vi "niFPGA Sine Wave Generator.vi"(1 "reset":bool) -> (4 "sine out":i16)   [LabVIEW 2017]
doc: "Generates a point-by-point sine wave using direct digital synthesis. The synthesis runs continuously from the top-level FPGA target clock to produce an accurate real-time frequency. Each execution of this VI returns the most recent sample produced by the underlying synthesis engine."
panel:
  out "cosine out":i16
  in  "phase offset (periods)":fxp<+,32,0>
  in  "frequency (periods/tick)":fxp<+,32,0>=0.9999999997671694
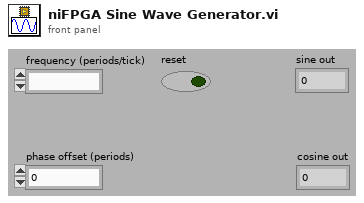
[diagram p1: front panel]
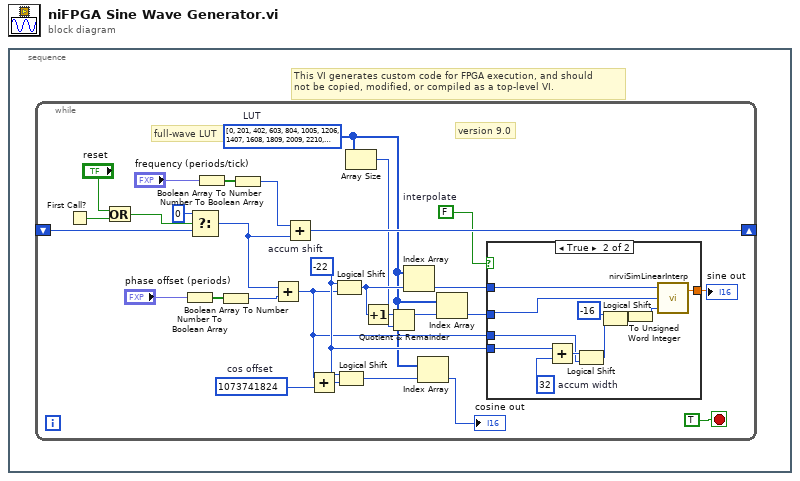
[diagram p0: block diagram]
diagram:
  n1 = stacked-sequence {
    frame #0 {
      # "This VI generates custom code for FPGA execution, and should\nnot be copied, modified, or compiled as a top-level VI."
      n2 = while {
        shift-right: [w28] -> _
        shift-left: _ -> [w18]
        stop <- TRUE stop-if-true
        w1 = u32 1073741824  # cos offset
        w8 = i32[] [0, 201, 402, 603, 804, 1005, 1206, 1407, 1608, 1809, 2009, 2210, 2411, 2611, 2811, 3012, 3212, 3412, 3612, 3811, 4011, 4211, 4410, 4609, 4808, 5007, 5205, 5404, 5602, 5800, 5998, 6195, 6393, 6590, 6787, 6983, 7179, 7375, 7571, 7767, 7962, 8157, 8351, 8546, 8740, 8933, 9126, 9319, 9512, 9704, 9896, 10087, 10279, 10469, 10660, 10850, 11039, 11228, 11417, 11605, 11793, 11980, 12167, 12354, 12540, 12725, 12910, 13095, 13279, 13462, 13645, 13828, 14010, 14191, 14372, 14553, 14733, 14912, 15091, 15269, 15446, 15624, 15800, 15976, 16151, 16326, 16500, 16673, 16846, 17018, 17189, 17360, 17531, 17700, 17869, 18037, 18205, 18371, 18538, 18703, 18868, 19032, 19195, 19358, 19520, 19681, 19841, 20001, 20160, 20318, 20475, 20632, 20787, 20943, 21097, 21250, 21403, 21555, 21706, 21856, 22005, 22154, 22302, 22448, 22595, 22740, 22884, 23028, 23170, 23312, 23453, 23593, 23732, 23870, 24007, 24144, 24279, 24414, 24547, 24680, 24812, 24943, 25073, 25202, 25330, 25457, 25583, 25708, 25832, 25955, 26078, 26199, 26319, 26438, 26557, 26674, 26790, 26905, 27020, 27133, 27245, 27356, 27467, 27576, 27684, 27791, 27897, 28002, 28106, 28208, 28310, 28411, 28511, 28609, 28707, 28803, 28898, 28993, 29086, 29178, 29269, 29359, 29447, 29535, 29621, 29707, 29791, 29874, 29956, 30037, 30117, 30196, 30273, 30350, 30425, 30499, 30572, 30644, 30714, 30784, 30852, 30919, 30985, 31050, 31114, 31176, 31237, 31298, 31357, 31414, 31471, 31526, 31581, 31634, 31685, 31736, 31785, 31834, 31881, 31927, 31971, 32015, 32057, 32098, 32138, 32177, 32214, 32250, 32285, 32319, 32351, 32383, 32413, 32442, 32469, 32496, 32521, 32545, 32568, 32589, 32610, 32629, 32647, 32663, 32679, 32693, 32706, 32718, 32728, 32737, 32745, 32752, 32758, 32762, 32765, 32767, 32767, 32767, 32765, 32762, 32758, 32752, 32745, 32737, 32728, 32718, 32706, 32693, 32679, 32663, 32647, 32629, 32610, 32589, 32568, 32545, 32521, 32496, 32469, 32442, 32413, 32383, 32351, 32319, 32285, 32250, 32214, 32177, 32138, 32098, 32057, 32015, 31971, 31927, 31881, 31834, 31785, 31736, 31685, 31634, 31581, 31526, 31471, 31414, 31357, 31298, 31237, 31176, 31114, 31050, 30985, 30919, 30852, 30784, 30714, 30644, 30572, 30499, 30425, 30350, 30273, 30196, 30117, 30037, 29956, 29874, 29791, 29707, 29621, 29535, 29447, 29359, 29269, 29178, 29086, 28993, 28898, 28803, 28707, 28609, 28511, 28411, 28310, 28208, 28106, 28002, 27897, 27791, 27684, 27576, 27467, 27356, 27245, 27133, 27020, 26905, 26790, 26674, 26557, 26438, 26319, 26199, 26078, 25955, 25832, 25708, 25583, 25457, 25330, 25202, 25073, 24943, 24812, 24680, 24547, 24414, 24279, 24144, 24007, 23870, 23732, 23593, 23453, 23312, 23170, 23028, 22884, 22740, 22595, 22448, 22302, 22154, 22005, 21856, 21706, 21555, 21403, 21250, 21097, 20943, 20787, 20632, 20475, 20318, 20160, 20001, 19841, 19681, 19520, 19358, 19195, 19032, 18868, 18703, 18538, 18371, 18205, 18037, 17869, 17700, 17531, 17360, 17189, 17018, 16846, 16673, 16500, 16326, 16151, 15976, 15800, 15624, 15446, 15269, 15091, 14912, 14733, 14553, 14372, 14191, 14010, 13828, 13645, 13462, 13279, 13095, 12910, 12725, 12540, 12354, 12167, 11980, 11793, 11605, 11417, 11228, 11039, 10850, 10660, 10469, 10279, 10087, 9896, 9704, 9512, 9319, 9126, 8933, 8740, 8546, 8351, 8157, 7962, 7767, 7571, 7375, 7179, 6983, 6787, 6590, 6393, 6195, 5998, 5800, 5602, 5404, 5205, 5007, 4808, 4609, 4410, 4211, 4011, 3811, 3612, 3412, 3212, 3012, 2811, 2611, 2411, 2210, 2009, 1809, 1608, 1407, 1206, 1005, 804, 603, 402, 201, 0, -201, -402, -603, -804, -1005, -1206, -1407, -1608, -1809, -2009, -2210, -2411, -2611, -2811, -3012, -3212, -3412, -3612, -3811, -4011, -4211, -4410, -4609, -4808, -5007, -5205, -5404, -5602, -5800, -5998, -6195, -6393, -6590, -6787, -6983, -7179, -7375, -7571, -7767, -7962, -8157, -8351, -8546, -8740, -8933, -9126, -9319, -9512, -9704, -9896, -10087, -10279, -10469, -10660, -10850, -11039, -11228, -11417, -11605, -11793, -11980, -12167, -12354, -12540, -12725, -12910, -13095, -13279, -13462, -13645, -13828, -14010, -14191, -14372, -14553, -14733, -14912, -15091, -15269, -15446, -15624, -15800, -15976, -16151, -16326, -16500, -16673, -16846, -17018, -17189, -17360, -17531, -17700, -17869, -18037, -18205, -18371, -18538, -18703, -18868, -19032, -19195, -19358, -19520, -19681, -19841, -20001, -20160, -20318, -20475, -20632, -20787, -20943, -21097, -21250, -21403, -21555, -21706, -21856, -22005, -22154, -22302, -22448, -22595, -22740, -22884, -23028, -23170, -23312, -23453, -23593, -23732, -23870, -24007, -24144, -24279, -24414, -24547, -24680, -24812, -24943, -25073, -25202, -25330, -25457, -25583, -25708, -25832, -25955, -26078, -26199, -26319, -26438, -26557, -26674, -26790, -26905, -27020, -27133, -27245, -27356, -27467, -27576, -27684, -27791, -27897, -28002, -28106, -28208, -28310, -28411, -28511, -28609, -28707, -28803, -28898, -28993, -29086, -29178, -29269, -29359, -29447, -29535, -29621, -29707, -29791, -29874, -29956, -30037, -30117, -30196, -30273, -30350, -30425, -30499, -30572, -30644, -30714, -30784, -30852, -30919, -30985, -31050, -31114, -31176, -31237, -31298, -31357, -31414, -31471, -31526, -31581, -31634, -31685, -31736, -31785, -31834, -31881, -31927, -31971, -32015, -32057, -32098, -32138, -32177, -32214, -32250, -32285, -32319, -32351, -32383, -32413, -32442, -32469, -32496, -32521, -32545, -32568, -32589, -32610, -32629, -32647, -32663, -32679, -32693, -32706, -32718, -32728, -32737, -32745, -32752, -32758, -32762, -32765, -32767, -32767, -32767, -32765, -32762, -32758, -32752, -32745, -32737, -32728, -32718, -32706, -32693, -32679, -32663, -32647, -32629, -32610, -32589, -32568, -32545, -32521, -32496, -32469, -32442, -32413, -32383, -32351, -32319, -32285, -32250, -32214, -32177, -32138, -32098, -32057, -32015, -31971, -31927, -31881, -31834, -31785, -31736, -31685, -31634, -31581, -31526, -31471, -31414, -31357, -31298, -31237, -31176, -31114, -31050, -30985, -30919, -30852, -30784, -30714, -30644, -30572, -30499, -30425, -30350, -30273, -30196, -30117, -30037, -29956, -29874, -29791, -29707, -29621, -29535, -29447, -29359, -29269, -29178, -29086, -28993, -28898, -28803, -28707, -28609, -28511, -28411, -28310, -28208, -28106, -28002, -27897, -27791, -27684, -27576, -27467, -27356, -27245, -27133, -27020, -26905, -26790, -26674, -26557, -26438, -26319, -26199, -26078, -25955, -25832, -25708, -25583, -25457, -25330, -25202, -25073, -24943, -24812, -24680, -24547, -24414, -24279, -24144, -24007, -23870, -23732, -23593, -23453, -23312, -23170, -23028, -22884, -22740, -22595, -22448, -22302, -22154, -22005, -21856, -21706, -21555, -21403, -21250, -21097, -20943, -20787, -20632, -20475, -20318, -20160, -20001, -19841, -19681, -19520, -19358, -19195, -19032, -18868, -18703, -18538, -18371, -18205, -18037, -17869, -17700, -17531, -17360, -17189, -17018, -16846, -16673, -16500, -16326, -16151, -15976, -15800, -15624, -15446, -15269, -15091, -14912, -14733, -14553, -14372, -14191, -14010, -13828, -13645, -13462, -13279, -13095, -12910, -12725, -12540, -12354, -12167, -11980, -11793, -11605, -11417, -11228, -11039, -10850, -10660, -10469, -10279, -10087, -9896, -9704, -9512, -9319, -9126, -8933, -8740, -8546, -8351, -8157, -7962, -7767, -7571, -7375, -7179, -6983, -6787, -6590, -6393, -6195, -5998, -5800, -5602, -5404, -5205, -5007, -4808, -4609, -4410, -4211, -4011, -3811, -3612, -3412, -3212, -3012, -2811, -2611, -2411, -2210, -2009, -1809, -1608, -1407, -1206, -1005, -804, -603, -402, -201]  # LUT
        w21 = FALSE  # interpolate
        w20 = i8 -22  # accum shift
        # "version 9.0"
        # "full-wave LUT"
        n3 = First Call?() -> (First Call?: T/F=w16:bool)
        n4 = Or(x="reset", y=w16) -> (x .or. y?=w15:bool)
        n5 = Number To Boolean Array(number="phase offset (periods)") -> (Boolean array=w4:bool[])
        n6 = Select(t=u32 0, s=w15, f=w18) -> (s? t:f=w26:u32)
        n7 = Number To Boolean Array(number="frequency (periods/tick)") -> (Boolean array=w7:bool[])
        n8 = Boolean Array To Number(Boolean array=w4) -> (number=w2:u32)
        n9 = Boolean Array To Number(Boolean array=w7) -> (number=w5:u32)
        n10 = Add(x=w26, y=w2) -> (x+y=w19:u32)
        n11 = Add(x=w5, y=w26) -> (x+y=w28:u32)
        n12 = Add(x=w19, y=w1) -> (x+y=w25:u32)
        n13 = Logical Shift(y=w20, x=w19) -> (x << y=w13:u32)
        n14 = Logical Shift(y=w20, x=w25) -> (x << y=w24:u32)
        n15 = Array Size(array=w8) -> (size(s)=w9:i32)
        n16 = Increment(x=w13) -> (x+1=w14:u32)
        n17 = Quotient & Remainder(x=w14, y=w9) -> (x-y*floor(x/y)=w11:u32)  [unwired: 1 out]
        n18 = Index Array(array=w8, index=w13) -> (element=w12:i32)
        n19 = Index Array(array=w8, index=w24) -> (element=→"cosine out":i32)
        n20 = Index Array(array=w8, index=w11) -> (element=w10:i32)
        n21 = case shown="True" w21 {
          tunnel: w12 -> [w30 w32]
          tunnel: [w30 w31] -> w22
          tunnel: w20 -> [_ w41]
          tunnel: w19 -> [_ w38]
          tunnel: w10 -> [_ w33]
          frame False {
          }
          frame True {
            w40 = i8 32  # accum width
            n22 = Add(x=w41, y=w40) -> (x+y=w39:i8)
            n23 = Logical Shift(y=w39, x=w38) -> (x << y=w37:u32)
            n24 = Logical Shift(y=-16, x=w37) -> (x << y=w35:u32)
            n25 = To Unsigned Word Integer(number=w35) -> (unsigned 16bit integer=w34:u16)
            n26 = call <vilib>:"nirviSimLinearInterp.vi"("y0"=w32, "y1"=w33, "x (fractional)"=w34) -> ("y"=w31:dbl)  [unwired: 6 out]
          }
        }
        "sine out" <- w22
      }
    }
  }
